vi "img.jpg.Write.pix.u8.vi"(8 "error in":errorcluster, 10 "pix.u8":u8[][](array[numeric]), 11 "path":path) -> (0 "error out":errorcluster)   [LabVIEW 2020]
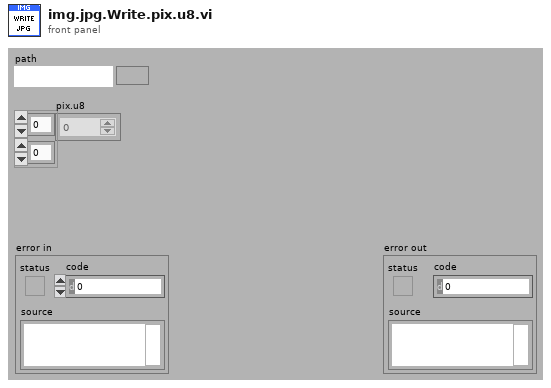
[diagram p1: front panel]
types:
  T1 = typedef "imagedata.ctl" = cluster{"image type":i32, "image depth":i32, "image":u8[], "mask":u8[], "colors":u32[], "Rectangle":cluster{"left":i16, "top":i16, "right":i16, "bottom":i16}}
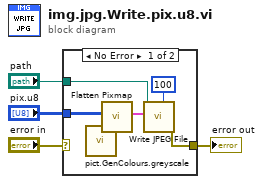
[diagram p0: block diagram]
diagram:
  n1 = case shown="No Error" "error in" {
    selector: "error in" -> [_ w11]
    tunnel: "pix.u8" -> [w10 _]
    tunnel: "path" -> [w8 _]
    tunnel: [w7 w11] -> w2
    frame No Error {
      n2 = call "pict.GenColours.greyscale.vi"() -> ("colours"=w5:u32[])  [unwired: 11 in]
      n3 = call <vilib>:"Flatten Pixmap.vi"("colors"=w5, "8-bit pixmap"=w10) -> ("image data"=w9:T1)  [unwired: 4 in, 5 out]
      n4 = call <vilib>:"Write JPEG File.vi"("quality (80)"=100, "image data"=w9, "path to JPEG file"=w8) -> ("error out"=w7:errorcluster)  [unwired: 7 in, 1 out]
    }
    frame Error {
    }
  }
  "error out" <- w2
